vi "Prepare Stream.vi"(8 "error in (no error)":errorcluster, 10 "Stream In":refnum<class "Stream.lvclass">, 11 "Endpoint in":refnum<class "Endpoint.lvclass">) -> (0 "error out":errorcluster, 2 "Stream":refnum<class "Stream.lvclass">, 3 "Endpoint out":refnum<class "Endpoint.lvclass">)   [LabVIEW 2020, in "Stream.lvlib" / "Endpoint.lvclass"]
uses:
  Endpoint.lvclass
  Stream/Stream.lvclass
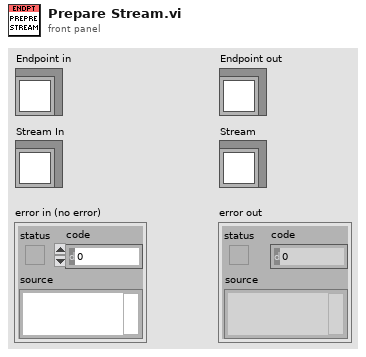
[diagram p1: front panel]
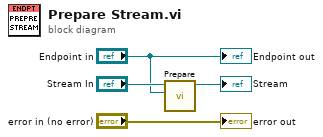
[diagram p0: block diagram]
diagram:
  n1 = call "Prepare.vi"("Endpoint"="Endpoint in", "Stream in"="Stream In") -> ("Stream out"=→"Stream":refnum<class "Stream.lvclass">)  [unwired: 8 in, 1 out]
  "error out" <- "error in (no error)"
  "Endpoint out" <- "Endpoint in"
